vi "Instrument Status Checking.vi"(8 "error in (no error)":errorcluster, 9 "Status Checking (On)":bool=TRUE, 11 "VISA resource name":refnum<visa-resource-name>) -> (0 "error out":errorcluster, 3 "VISA resource name out":refnum<visa-resource-name>)   [LabVIEW 2020, in "Rohde&Schwarz CMXP GPRF.lvlib"]
doc: "This VI switches state checking of the instrument driver (*STB? query bit 2). Subsequently, all the driver VIs are using the state checking to immediately react on error that might have occured. We recommend to keep the state checking ON all the time. Switch it OFF only in rare cases when you require maximum speed.\nThe default state after initializing the session is <b>ON</b>."
uses:
  <instrlib>/Rohde&Schwarz CMXP GPRF/Rohde&Schwarz CMXP GPRF.lvlib
  <instrlib>/Rohde&Schwarz CMXP GPRF/Private/rsidr_core.llb/type_Session_Parameter_Boolean.ctl
  <instrlib>/Rohde&Schwarz CMXP GPRF/Private/rsidr_core.llb/rsidr_core.lvlib
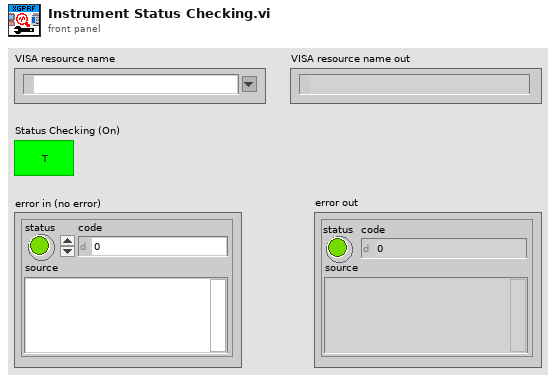
[diagram p1: front panel]
types:
  T1 = typedef "Rohde&Schwarz CMXP GPRF.lvlib/rsidr_core.lvlib/type_Session_Parameter_Boolean.ctl" = enum16{"Simulate", "Query Instr Status", "Check Range", "Check Options", "Add LF to Write", "Duplicate Session", "Fast Sweep", "Logging", "OPC-sync Attribute Queries", "OPC-sync Attribute Writes"}
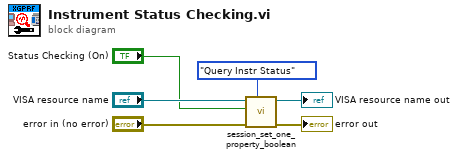
[diagram p0: block diagram]
diagram:
  n1 = call <instrlib>:"session_set_one_property_boolean.vi"("Session Parameter Boolean"=type_Session_Parameter_Boolean."Query Instr Status" ("Session Parameter boolean"), "error in"="error in (no error)", "Boolean value in"="Status Checking (On)", "VISA resource name"="VISA resource name") -> ("error out"=→"error out":errorcluster, "VISA resource name out"=→"VISA resource name out":refnum<visa-resource-name>)  [unwired: 5 in, 1 out]
